vi "functional global counter 1.vi"() -> ()   [LabVIEW 2009]
uses:
  Functional Global Command.ctl
panel:
  out "Compte 1":i32
  out "total cumulatif":i32
  in  "stop":bool
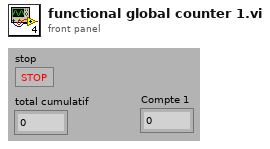
[diagram p1: front panel]
types:
  T1 = typedef "Functional Global Command.ctl" = enum16{"Réinitialiser", "Incrémenter", "Obtenir le compte"}
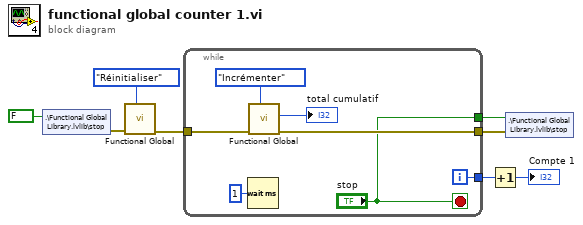
[diagram p0: block diagram]
diagram:
  n1 = shared-variable ".\\Functional Global Library.lvlib\\stop"(FALSE ("stop")) -> (error out=w2:errorcluster)  [unwired: 1 in]
  n2 = call "Functional Global.vi"("Commande"=Functional_Global_Command."Réinitialiser" ("Command"), "entrée d'erreur (pas d'erreur)"=w2) -> ("sortie d'erreur"=w5:errorcluster)  [unwired: 8 in, 1 out]
  n3 = while "Boucle While" {
    tunnel: [w15] -> w8
    tunnel: [w10] -> w4
    tunnel: w5 -> [w12]
    tunnel: ["stop"] -> w3
    i -> [w15]
    stop <- "stop" stop-if-true
    n4 = Wait (ms) ("Attendre (ms)")(milliseconds to wait=u32 1) -> ()  [unwired: 1 out]
    n5 = call "Functional Global.vi"("Commande"=Functional_Global_Command."Incrémenter" ("Command"), "entrée d'erreur (pas d'erreur)"=w12) -> ("sortie d'erreur"=w10:errorcluster, "Compte"=→"total cumulatif":i32)  [unwired: 8 in]
  }
  n6 = Increment ("Incrémenter")(x=w8) -> (x+1=→"Compte 1":i32)
  n7 = shared-variable ".\\Functional Global Library.lvlib\\stop"(w3, error in=w4) -> ()  [unwired: 1 out]
